vi "RSNRPZ Configure Statistics Timegate.vi"(5 "Time (0.01 s)":dbl=0.01 format="%^.3e", 6 "Midamble Length (0.0 s)":dbl format="%^.3e", 7 "Midamble Offset (0.0 s)":dbl format="%^.3e", 8 "error in (no error)":errorcluster, 9 "Offset (0.0 s)":dbl format="%^.3e", 10 "Channel (1)":i32=1, 11 "VISA session":refnum<visa-resource-name> caption="VISA resource name") -> (0 "error out":errorcluster, 3 "dup VISA session":refnum<visa-resource-name> caption="VISA resource name")   [LabVIEW 2010]
doc: "This VI configures the timegate (depends on trigger event) in which the sensor is doing statistic measurements.\n\nRemote-control command(s):\nSENSe:STATistics:OFFSet:TIME\nSENSe:STATistics:TIME\nSENSe:STATistics:[EXCLude]:MID:OFFSet[:TIME]\nSENSe:STATistics:[EXCLude]:MID:TIME"
uses:
  rsnrpz_32.dll
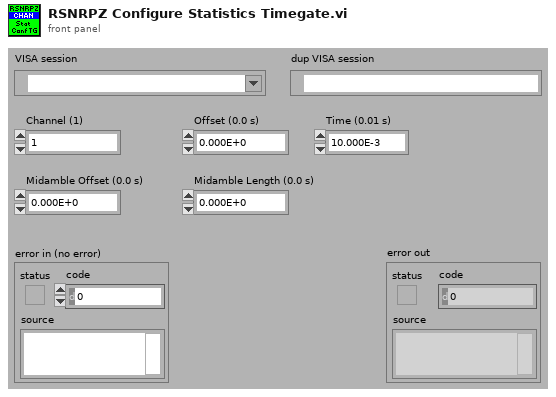
[diagram p1: front panel]
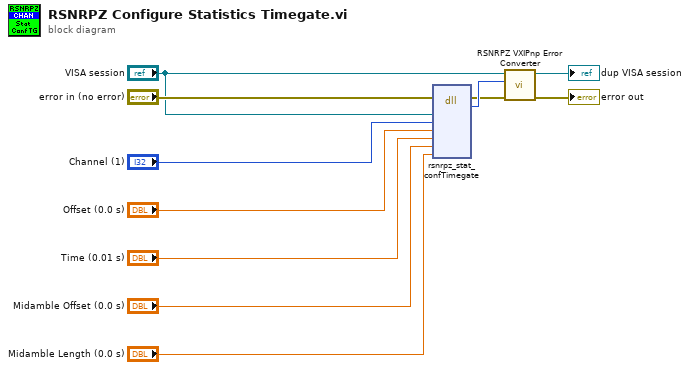
[diagram p0: block diagram]
diagram:
  n1 = dll-call lib="rsnrpz_32.dll" fn="rsnrpz_stat_confTimegate"(error in="error in (no error)", "Instrument Handle"="VISA session", "Channel"="Channel (1)", "Offset"="Offset (0.0 s)", "Time"="Time (0.01 s)", "Midamble Offset"="Midamble Offset (0.0 s)", "Midamble Length"="Midamble Length (0.0 s)") -> (error out=w5:errorcluster, "Status"=w11:i32)  [unwired: 8 in, 1 out]
  n2 = call <instrlib>:"RSNRPZ VXIPnp Error Converter.vi"("error in"=w5, "VXIPnp error code"=w11, "VISA session"="VISA session") -> ("error out"=→"error out":errorcluster, "dup VISA session"=→"dup VISA session":refnum<visa-resource-name>)  [unwired: 7 in]
